vi "from_STR_to_PLC_STRING[30].vi"(8 "error_in":errorcluster, 11 "String":string) -> (0 "error_out":errorcluster, 3 "byte_array":u8[](array[numeric]))   [LabVIEW 2020]
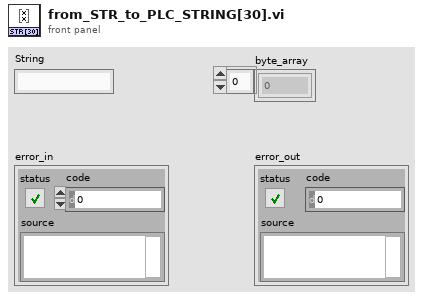
[diagram p1: front panel]
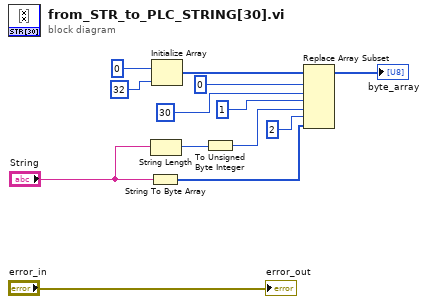
[diagram p0: block diagram]
diagram:
  n1 = String To Byte Array(string="String") -> (unsigned byte array=w3:u8[])
  n2 = String Length(string="String") -> (length=w5:i32)
  n3 = Initialize Array(u8 0, 32 ("dimension size")) -> (w10:u8[])
  n4 = To Unsigned Byte Integer(number=w5) -> (unsigned 8bit integer=w4:u8)
  n5 = Replace Array Subset(array=w10, new element #1=u8 30, index #1=0 ("index"), new element #2=w4, index #2=1 ("index"), new element #3=w3, index #3=2 ("index")) -> (→"byte_array":u8[])
  "error_out" <- "error_in"
